vi "System_Test_Initialize Tags.vi"() -> ()   [LabVIEW 2015, in "System.lvclass"]
uses:
  System.lvclass
  <vilib>/NI/Tag Bus/tag/tag descriptor.lvclass/tag descriptor.ctl
  <vilib>/NI/Tag Bus/tag/tag descriptor.lvclass
panel:
  out "Tag Names":string[](array[string])
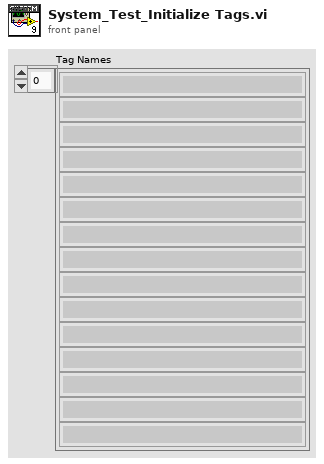
[diagram p1: front panel]
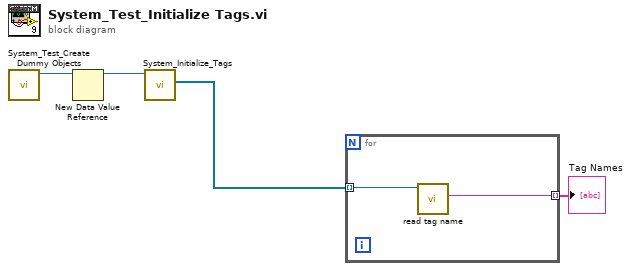
[diagram p0: block diagram]
diagram:
  n1 = call "System_Test_Create Dummy Objects.vi"() -> ("System.lvclass"=w2:refnum<class "System.lvclass">)  [unwired: 10 in, 1 out]
  n2 = New Data Value Reference(data value=w2) -> (data value reference=w1:refnum<data-value>)  [unwired: 1 in, 1 out]
  n3 = call "System_Initialize_Tags.vi"("System DVR"=w1) -> ("TagDescriptions"=w4:refnum<class "tag descriptor.lvclass">[])  [unwired: 8 in, 2 out]
  n4 = for {
    tunnel: w4 -> [w6] mode=indexing
    tunnel: [w5] -> w3 mode=indexing
    n5 = call <vilib>:"read tag name.vi"("system tag in"=w6) -> ("name"=w5:string)  [unwired: 8 in, 2 out]
  }
  "Tag Names" <- w3
